vi "Emergency stop.vi"(8 "error in":errorcluster) -> (0 "error out":errorcluster)   [LabVIEW 2011]
panel:
  # "Emergency stop the motion server.  This can only be reset  by restarting the server."
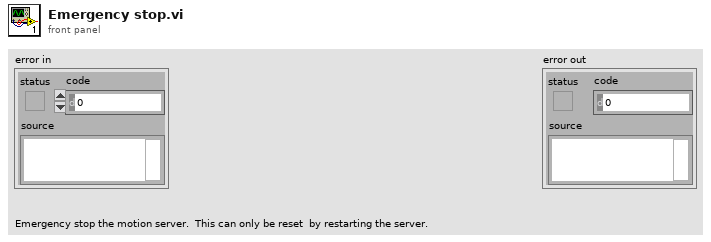
[diagram p1: front panel]
types:
  T1 = typedef "motion_variables.ctl" = cluster{"Motion command":refnum<k21>, "Motion status":refnum<k21>, "Emergency stop":refnum<k21>}
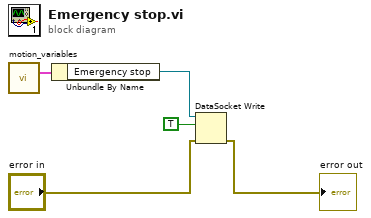
[diagram p0: block diagram]
diagram:
  n1 = call "motion_variables.vi"() -> ("Motion variables"=w5:T1)  [unwired: 11 in]
  n2 = Unbundle By Name(w5) -> ("Emergency stop"=w4:refnum<k21>)
  n3 = DataSocket Write(8:"error in", 10:TRUE ("timed out"), 11:w4) -> (0:→"error out":errorcluster)  [unwired: 1 in, 2 out]
